vi "intIntToString.vi"(8 "Error in (no error)":errorcluster, 11 "Int in":refnum<class "IntClass.lvclass">) -> (0 "Error out":errorcluster, 1 "String format":T1=10 items=["Binary"=2, "Octal"=8, "Decimal"=10, "Hexadecimal"=16, "Hexatrigesimal"=36, "ASCII"=64], 2 "String":string, 3 "Int out":refnum<class "IntClass.lvclass">)   [LabVIEW 2011, in "IntClass.lvclass"]
uses:
  IntClass.lvclass
  UintClass/enumBase.ctl
  IntClass.lvclass/IntClass.ctl
  UintClass/UintClass.lvclass
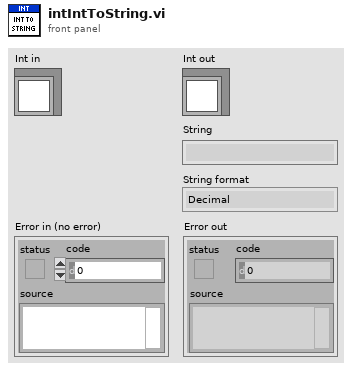
[diagram p1: front panel]
types:
  T1 = typedef "UintClass.lvclass/enumBase.ctl" = u16
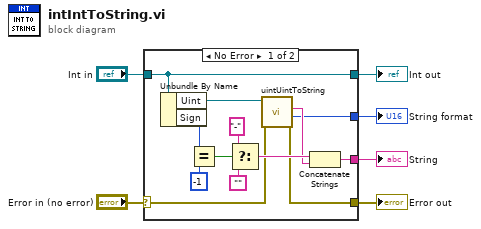
[diagram p0: block diagram]
diagram:
  n1 = case shown="No Error" "Error in (no error)" {
    selector: "Error in (no error)" -> [w11 w21]
    tunnel: [w10 w21] -> w6
    tunnel: [w19 w20] -> w3
    tunnel: "Int in" -> [w19 w20]
    tunnel: [w8 _] -> w2
    tunnel: [w7 _] -> w1
    frame No Error {
      n2 = Unbundle By Name(w19) -> ("Uint"=w12:refnum<class "UintClass.lvclass">, "Sign"=w18:i8)
      n3 = Equal?(x=w18, y=i8 -1) -> (x = y?=w16:bool)
      n4 = Select(t="-", s=w16, f="") -> (s? t:f=w13:string)
      n5 = call "uintUintToString.vi"("Error in (no error)"=w11, "Uint in"=w12) -> ("Error out"=w10:errorcluster, "String format (decimal)"=w8:T1, "String"=w9:string)  [unwired: 6 in, 1 out]
      n6 = Concatenate Strings(w13, w9) -> (w7:string)
    }
    frame Error {
    }
  }
  "Int out" <- w3
  "Error out" <- w6
  "String format" <- w2
  "String" <- w1
